vi "AlliGator Parse Python Function Input Parameters.vi"(8 "Error In":errorcluster, 9 "Source":string, 11 "Input String":string) -> (0 "Error Out":errorcluster, 1 "Function Input Parameters":T1[](array[typedef]), 3 "Output string":string)   [LabVIEW 2021, in "AlliGator Python Plugins.lvlib"]
doc: "Looks for Python Plugin Input Paramater Section Header and Footer and returns the parameter names, types and descriptions\n\nIf the section is found, the part that follows that section is returned."
uses:
  AlliGator Python Plugins.lvlib
  AlliGator Python Function Parameter Definition.ctl
  Strings/Strings.lvlib
panel:
  # "see the AlliGator License on the block diagram (Ctrl+E or Window:Show Block Diagram)"
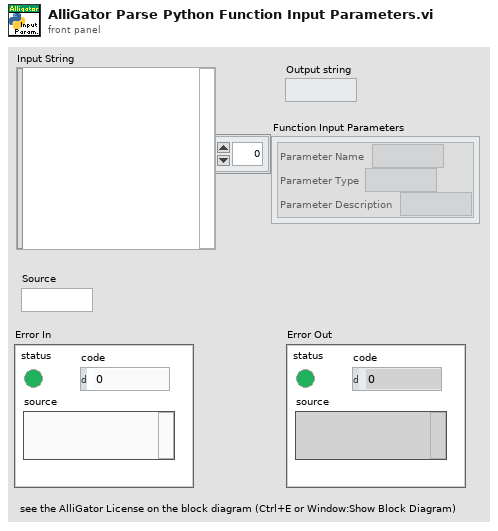
[diagram p1: front panel]
types:
  T1 = typedef "AlliGator Python Plugins.lvlib/AlliGator Python Function Parameter Definition.ctl" = cluster{"Parameter Name":string, "Parameter Type":string, "Parameter Description":string}
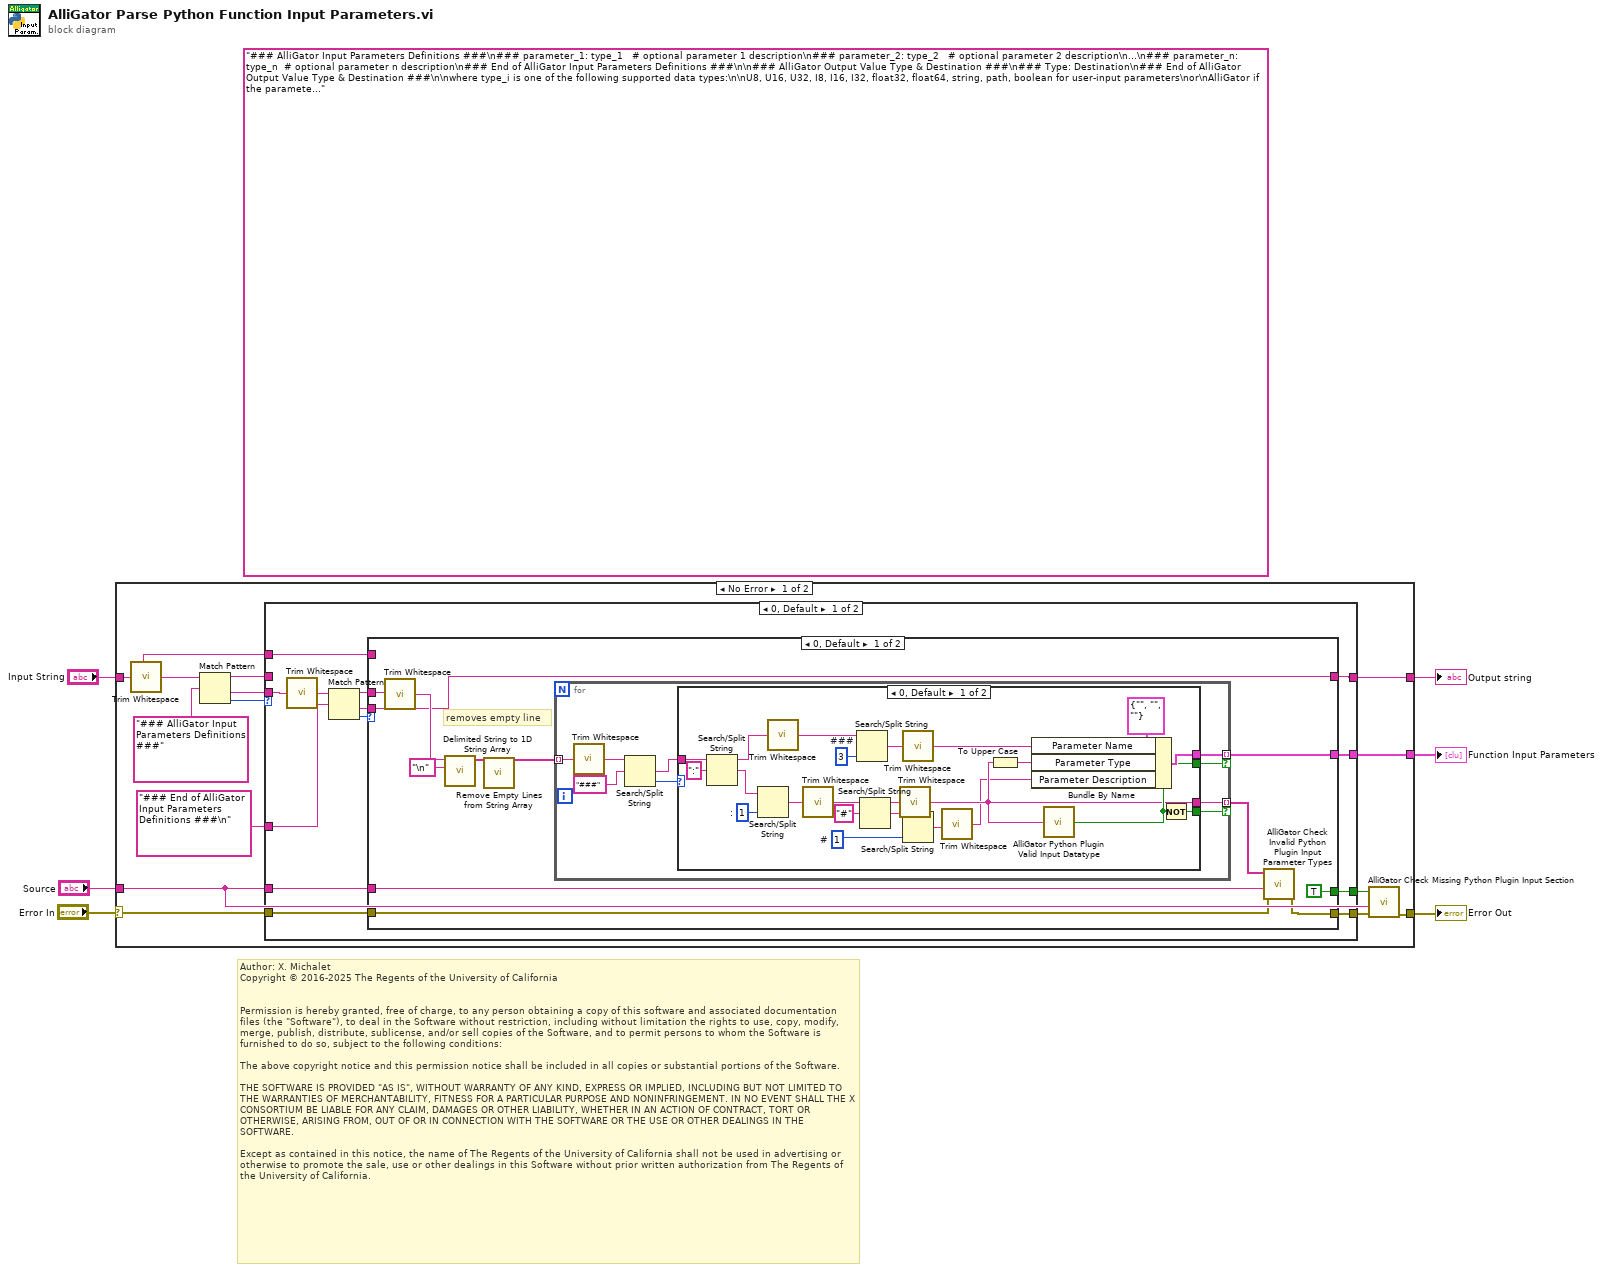
[diagram p0: block diagram]
diagram:
  (unwired) "### AlliGator Input Parameters Definitions ###\n### parameter_1: type_1   # optional parameter 1 description\n### parameter_2: type_2   # optional parameter 2 description\n...\n### parameter_n: type_n  # optional parameter n description\n### End of AlliGator Input Parameters Definitions ###\n\n### AlliGator Output Value Type & Destination ###\n### Type: Destination\n### End of AlliGator Output Value Type & Destination ###\n\nwhere type_i is one of the following supported data types:\n\nU8, U16, U32, I8, I16, I32, float32, float64, string, path, boolean for user-input parameters\nor\nAlliGator if the parameter is an internal one (in which case parameter_i needs to match the internal parameter's name exactly)\n\nSupported output value_type are:\n\nplot, image, FLI dataset\n\nSupportef output destinations are:\n\ndecay graph, image sum, image max, image mask, white light image, FLI dataset"
  # "Author: X. Michalet\nCopyright © 2016-2025 The Regents of the University of California\n \n\nPermission is hereby granted, free of charge, to any person obtaining a copy of this software and associated documentation files (the \"Software\"), to deal in the Software without restriction, including without limitation the rights to use, copy, modify, merge, publish, distribute, sublicense, and/or sell copies of the Software, and to permit persons to whom the Software is furnished to do so, subject to the following conditions:\n\nThe above copyright notice and this permission notice shall be included in all copies or substantial portions of the Software.\n\nTHE SOFTWARE IS PROVIDED \"AS IS\", WITHOUT WARRANTY OF ANY KIND, EXPRESS OR IMPLIED, INCLUDING BUT NOT LIMITED TO THE WARRANTIES OF MERCHANTABILITY, FITNESS FOR A PARTICULAR PURPOSE AND NONINFRINGEMENT. IN NO EVENT SHALL THE X CONSORTIUM BE LIABLE FOR ANY CLAIM, DAMAGES OR OTHER LIABILITY, WHETHER IN AN ACTION OF CONTRACT, TORT OR OTHERWISE, ARISING FROM, OUT OF OR IN CONNECTION WITH THE SOFTWARE OR THE USE OR OTHER DEALINGS IN THE SOFTWARE.\n\nExcept as contained in this notice, the name of The Regents of the University of California shall not be used in advertising or otherwise to promote the sale, use or other dealings in this Software without prior written authorization from The Regents of the University of California."
  n1 = case shown="No Error" "Error In" {
    selector: "Error In" -> [w15 w83]
    tunnel: [w19 _] -> w6
    tunnel: "Input String" -> [w8 w82]
    tunnel: [w13 w83] -> w3
    tunnel: [w16 w82] -> w2
    tunnel: "Source" -> [w7 _]
    frame No Error {
      n2 = call <vilib>:"Trim Whitespace.vi"("string"=w8) -> ("trimmed string"=w18:string)  [unwired: 1 in]
      n3 = Match Pattern(string=w18, regular expression="### AlliGator Input Parameters Definitions ###" ("search string/char (-)")) -> (before substring=w20:string, after substring=w10:string, offset past match=w17:i32)  [unwired: 1 in, 1 out]
      n4 = case shown="0, Default" w17 {
        tunnel: w20 -> [_ _]
        tunnel: [w33 _] -> w19
        tunnel: [w26 w80] -> w16
        tunnel: "### End of AlliGator Input Parameters Definitions ###\n" ("search string/char (-)") -> [w31 _]
        tunnel: [w30 w81] -> w12
        tunnel: w15 -> [w29 w81]
        tunnel: w7 -> [w28 _]
        tunnel: [w23 _] -> w14
        tunnel: w10 -> [w25 _]
        tunnel: w8 -> [w22 w80]
        frame 0, Default {
          n5 = call <vilib>:"Trim Whitespace.vi"("string"=w25) -> ("trimmed string"=w32:string)  [unwired: 1 in]
          n6 = Match Pattern(string=w32, regular expression=w31) -> (before substring=w24:string, after substring=w21:string, offset past match=w27:i32)  [unwired: 1 in, 1 out]
          n7 = case shown="0, Default" w27 {
            tunnel: [w44 _] -> w33
            tunnel: [w39 w79] -> w30
            tunnel: w29 -> [w38 w79]
            tunnel: w28 -> [w37 _]
            tunnel: [w35 w78] -> w26
            tunnel: w24 -> [w36 _]
            tunnel: [TRUE ("Input Section Found") _] -> w23
            tunnel: w22 -> [_ w78]
            tunnel: w21 -> [w35 _]
            frame 0, Default {
              # "removes empty line"
              n8 = call <vilib>:"Trim Whitespace.vi"("string"=w36) -> ("trimmed string"=w41:string)  [unwired: 1 in]
              n9 = call <vilib>:"Delimited String to 1D String Array.vi"("delimiter"="\n", "delimited string"=w41) -> ("string array"=w43:string[])  [unwired: 9 in]
              n10 = call "Remove Empty Lines from String Array.vi"("string array in"=w43) -> ("string array out"=w42:string[])
              n11 = for {
                tunnel: w42 -> [w53] mode=indexing
                tunnel: [w54] -> w44 mode=indexing if=w52
                tunnel: [w50] -> w40 mode=indexing if=w51
                n12 = call <vilib>:"Trim Whitespace.vi"("string"=w53) -> ("trimmed string"=w49:string)  [unwired: 1 in]
                n13 = Search/Split String(string=w49, search string/char (-)="###") -> (match + rest of string=w48:string, offset of match=w46:i32)  [unwired: 1 in, 1 out]
                n14 = case shown="0, Default" w46 {
                  tunnel: [w77 _] -> w54
                  tunnel: [w72 _] -> w52
                  tunnel: [w71 _] -> w51
                  tunnel: [w67 _] -> w50
                  tunnel: w48 -> [w60 _]
                  frame 0, Default {
                    w57 = 1  # #
                    w73 = 3  # ###
                    w74 = 1  # :
                    n15 = Search/Split String(string=w60, search string/char (-)=":") -> (substring before match=w65:string, match + rest of string=w75:string)  [unwired: 1 in, 1 out]
                    n16 = Search/Split String(string=w75, offset (0)=w74) -> (match + rest of string=w69:string)  [unwired: 1 in, 2 out]
                    n17 = call <vilib>:"Trim Whitespace.vi"("string"=w65) -> ("trimmed string"=w66:string)  [unwired: 1 in]
                    n18 = call <vilib>:"Trim Whitespace.vi"("string"=w69) -> ("trimmed string"=w63:string)  [unwired: 1 in]
                    n19 = Search/Split String(string=w66, offset (0)=w73) -> (match + rest of string=w64:string)  [unwired: 1 in, 2 out]
                    n20 = Search/Split String(string=w63, search string/char (-)="#") -> (substring before match=w68:string, match + rest of string=w58:string)  [unwired: 1 in, 1 out]
                    n21 = call <vilib>:"Trim Whitespace.vi"("string"=w68) -> ("trimmed string"=w67:string)  [unwired: 1 in]
                    n22 = call <vilib>:"Trim Whitespace.vi"("string"=w64) -> ("trimmed string"=w61:string)  [unwired: 1 in]
                    n23 = Search/Split String(string=w58, offset (0)=w57) -> (match + rest of string=w55:string)  [unwired: 1 in, 2 out]
                    n24 = call <vilib>:"Trim Whitespace.vi"("string"=w55) -> ("trimmed string"=w56:string)  [unwired: 1 in]
                    n25 = To Upper Case(1:w67) -> (0:w59:string)
                    n26 = Bundle By Name(cluster=T1 {"Parameter Name"="", "Parameter Type"="", "Parameter Description"=""} ("Function Parameters"), "Parameter Name"=w61, "Parameter Type"=w59, "Parameter Description"=w56) -> (w77:T1)
                    n27 = call "AlliGator Python Plugin Valid Input Datatype.vi"("Input Datatype"=w67) -> ("Valid Datatype?"=w72:bool)  [unwired: 8 in]
                    n28 = Not(x=w72) -> (.not. x?=w71:bool)
                  }
                  frame -1 {
                  }
                }
              }
              n29 = call "AlliGator Check Invalid Python Plugin Input Parameter Types.vi"("error in (no error)"=w38, "Source"=w37, "Invalid Parameter Types"=w40) -> ("error out"=w39:errorcluster)  [unwired: 8 in]
            }
            frame -1 {
            }
          }
        }
        frame -1 {
          # "No Input Parameters section"
        }
      }
      n30 = call "AlliGator Check Missing Python Plugin Input Section.vi"("error in (no error)"=w12, "Source"=w7, "Input Section Found"=w14) -> ("error out"=w13:errorcluster)  [unwired: 8 in]
    }
    frame Error {
    }
  }
  "Function Input Parameters" <- w6
  "Error Out" <- w3
  "Output string" <- w2
